vi "MyArm3D.vi"() -> ()   [LabVIEW 2024]
uses:
  <vilib>/Native 3D Graph/xcontrol/3DPC_SurfacePlot.xctl
  <vilib>/Utility/miscctls.llb/LV3DPointTypeDef.ctl
  <vilib>/Analysis/Matrix/Datatypes/RealMatrix.ctl
  <vilib>/Analysis/baseanly.llb/Real A x B.vi
  <vilib>/Analysis/NI_AALBase.lvlib
  <vilib>/Analysis/Matrix/NI_Matrix.lvlib
panel:
  out "3D Picture 2":refnum<vi>(3d-picture)
  in  "Array":T1(array[cluster])
  out "2D Picture":picture
  out "3D Graph":refnum<class "Base Datatype.lvclass">[](xcontrol)
  out "3D Picture":refnum<vi>(3d-picture)
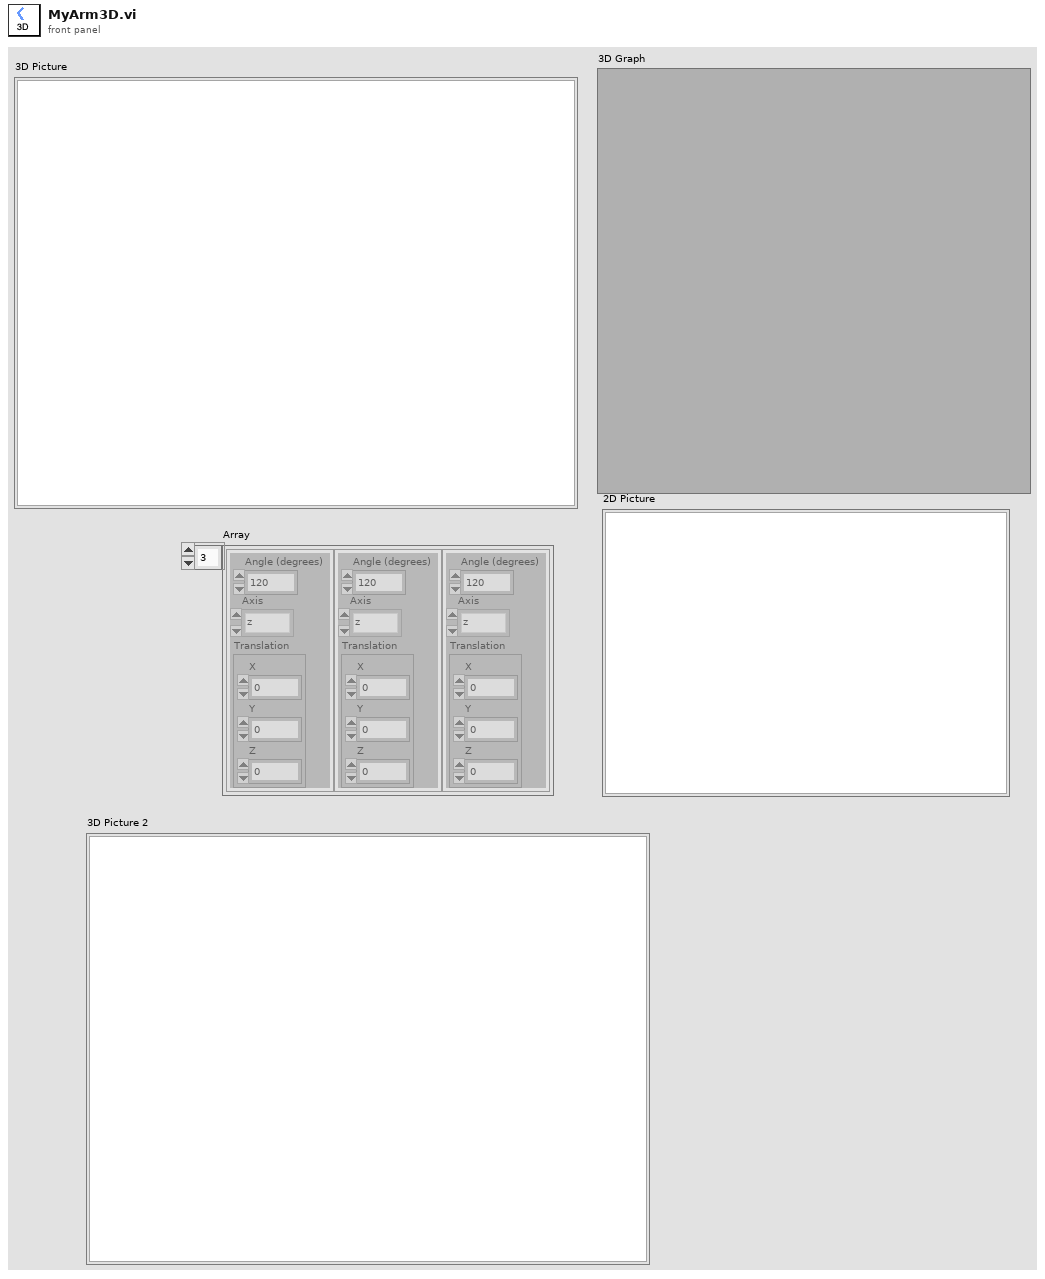
[diagram p1: front panel]
types:
  T1 = cluster{"Angle (degrees)":dbl, "Axis":enum16{"x", "y", "z"}, "Translation":cluster{"X":dbl, "Y":dbl, "Z":dbl}}[]
  T2 = typedef "NI_Matrix.lvlib/RealMatrix.ctl" = dbl[][]
  T3 = typedef "LV3DPointTypeDef.ctl" = cluster{"X":sgl, "Y":sgl, "Z":sgl}
  T4 = enum16{"None", "Spherical", "Flying", "Oriented"}
  T5 = cluster{"Line width":sgl, "Line Color":u32, "Axes?":bool}
  T6 = cluster{"Angle (degrees)":dbl, "Axis":enum16{"x", "y", "z"}, "Translation":cluster{"X":dbl, "Y":dbl, "Z":dbl}}
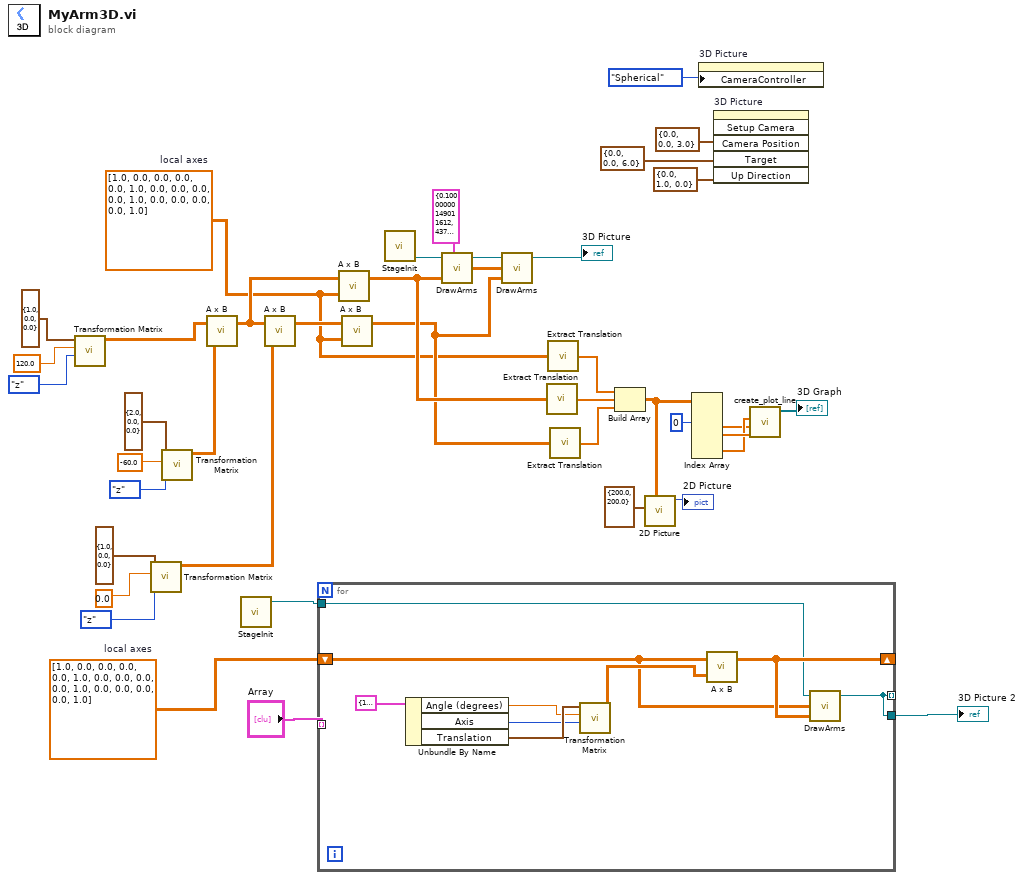
[diagram p0: block diagram]
diagram:
  w7 = T2 [[1.0, 0.0, 0.0, 0.0], [0.0, 1.0, 0.0, 0.0], [0.0, 0.0, 1.0, 0.0], [0.0, 0.0, 0.0, 1.0]]  # local axes
  w9 = T2 [[1.0, 0.0, 0.0, 0.0], [0.0, 1.0, 0.0, 0.0], [0.0, 0.0, 1.0, 0.0], [0.0, 0.0, 0.0, 1.0]]  # local axes
  n1 = call "Transformation Matrix.vi"("Axis"=enum16{"x", "y", "z"}."z", "Angle (degrees)"=120.0, "Translation"=cluster{"X":dbl, "Y":dbl, "Z":dbl} {"X"=1.0, "Y"=0.0, "Z"=0.0}) -> ("Transformation Matrix"=w1:T2)  [unwired: 8 in]
  n2 = call "Transformation Matrix.vi"("Axis"=enum16{"x", "y", "z"}."z", "Angle (degrees)"=0.0, "Translation"=cluster{"X":dbl, "Y":dbl, "Z":dbl} {"X"=1.0, "Y"=0.0, "Z"=0.0}) -> ("Transformation Matrix"=w26:T2)  [unwired: 8 in]
  n3 = call "Transformation Matrix.vi"("Axis"=enum16{"x", "y", "z"}."z", "Angle (degrees)"=-60.0, "Translation"=cluster{"X":dbl, "Y":dbl, "Z":dbl} {"X"=2.0, "Y"=0.0, "Z"=0.0}) -> ("Transformation Matrix"=w27:T2)  [unwired: 8 in]
  n4 = call-poly <vilib>:"A x B.vi"("B"=w27, "A"=w1) -> ("A x B"=w13:T2)  [unwired: 1 out]
  n5 = call "StageInit.vi"() -> ("Stage out"=w6:refnum<vi>)  [unwired: 4 in, 1 out]
  n6 = call-poly <vilib>:"A x B.vi"("B"=w26, "A"=w13) -> ("A x B"=w11:T2)  [unwired: 1 out]
  n7 = for {
    shift-right: [w45] -> _
    shift-left: w7 -> [w44]
    tunnel: "Array" -> [_] mode=indexing
    tunnel: w6 -> [w43]
    tunnel: [w42] -> _ mode=indexing
    tunnel: [w42] -> w5
    n8 = Unbundle By Name(T6 {"Angle (degrees)"=120.0, "Axis"=enum."z", "Translation"={"X"=0.0, "Y"=0.0, "Z"=0.0}}) -> ("Angle (degrees)"=w48:dbl, "Axis"=w47:enum16{"x", "y", "z"}, "Translation"=w49:cluster{"X":dbl, "Y":dbl, "Z":dbl})
    n9 = call "Transformation Matrix.vi"("Axis"=w47, "Angle (degrees)"=w48, "Translation"=w49) -> ("Transformation Matrix"=w46:T2)  [unwired: 8 in]
    n10 = call-poly <vilib>:"A x B.vi"("B"=w46, "A"=w44) -> ("A x B"=w45:T2)  [unwired: 1 out]
    n11 = call "DrawArms.vi"("Stage in"=w43, "Start"=w44, "End"=w45) -> ("Stage out"=w42:refnum<vi>)  [unwired: 3 in, 1 out]
  }
  "3D Picture 2" <- w5
  n12 = call-poly <vilib>:"A x B.vi"("B"=w9, "A"=w13) -> ("A x B"=w12:T2)  [unwired: 1 out]
  n13 = call-poly <vilib>:"A x B.vi"("B"=w9, "A"=w11) -> ("A x B"=w10:T2)  [unwired: 1 out]
  n14 = call "StageInit.vi"() -> ("Stage out"=w41:refnum<vi>)  [unwired: 4 in, 1 out]
  n15 = call "DrawArms.vi"("Stage in"=w41, "Params"=T5 {"Line width"=0.1, "Line Color"=4376575, "Axes?"=TRUE}, "End"=w12) -> ("Stage out"=w17:refnum<vi>, "End Out"=w15:T2)  [unwired: 3 in]
  n16 = call "DrawArms.vi"("Stage in"=w17, "Start"=w15, "End"=w10) -> ("Stage out"=→"3D Picture":refnum<vi>)  [unwired: 3 in, 1 out]
  n17 = call "Extract Translation.vi"("Transformation matrix"=w12) -> ("translation"=w24:dbl[])
  n18 = call "Extract Translation.vi"("Transformation matrix"=w9) -> ("translation"=w37:dbl[])
  n19 = call "Extract Translation.vi"("Transformation matrix"=w10) -> ("translation"=w23:dbl[])
  n20 = Build Array(w37, w24, w23) -> (w18:dbl[][])
  n21 = call "2D Picture.vi"("position array"=w18, "Origin"=cluster{"x":dbl, "y":dbl} {"x"=200.0, "y"=200.0}) -> ("picture out"=→"2D Picture":picture)  [unwired: 9 in]
  n22 = Index Array(array=w18, index (col) #1=0 ("disabled index (col)")) -> (element #1=w34:dbl[], element #2=w36:dbl[], element #3=w35:dbl[])  [unwired: 5 in]
  n23 = property on="3D Picture" class="SceneGraphDisp (strict)"("CameraController"=T4."Spherical" ("Camera Controller:Type")) -> ()  [unwired: 2 in, 2 out]
  n24 = invoke on="3D Picture" class="SceneGraphDisp (strict)" method="Setup Camera"("Camera Position"=T3 {"X"=0.0, "Y"=0.0, "Z"=6.0}, "Target"=T3 {"X"=0.0, "Y"=0.0, "Z"=3.0}, "Up Direction"=T3 {"X"=0.0, "Y"=1.0, "Z"=0.0}) -> ()  [unwired: 3 in, 6 out]
  n25 = call <vilib>:"create_plot_line.vi"("z vector"=w36, "y vector"=w34, "x vector"=w35) -> ("plots out"=→"3D Graph":refnum<class "Base Datatype.lvclass">[])  [unwired: 2 in, 6 out]
